vi "KlingerV2 ConvUnit.vi"   [LabVIEW 2019]
doc: "Ce VI convertit le nombre spécifié de l'unitée actuelle vers l'unité demandée. Les différentes unité de déplacement disponible sont les pas, les µm et les picosecondes."
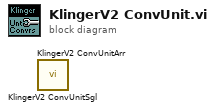
[diagram p0: block diagram]
diagram:
  n1 = call <userlib>:"KlingerV2 ConvUnitSgl.vi"() -> ()  [unwired: 14 in, 2 out]
  n2 = call <userlib>:"KlingerV2 ConvUnitArr.vi"() -> ()  [unwired: 14 in, 2 out]
